vi "Can Edit Cell.vi"(0 "State":T1, 7 "Cell":T6, 11 "NumRows":i32) -> (4 "locked":bool, 8 "can edit?":bool)   [LabVIEW 2020, in "KTable.xctl"]
uses:
  KTable.xctl
  <vilib>/Utility/miscctls.llb/LVRowAndColumnTypeDef.ctl
  State.ctl
  ColumnSpec.ctl
  ColumnType.ctl
  Table Properties.ctl
  Events.ctl
  Event Data.ctl
  Event Type.ctl
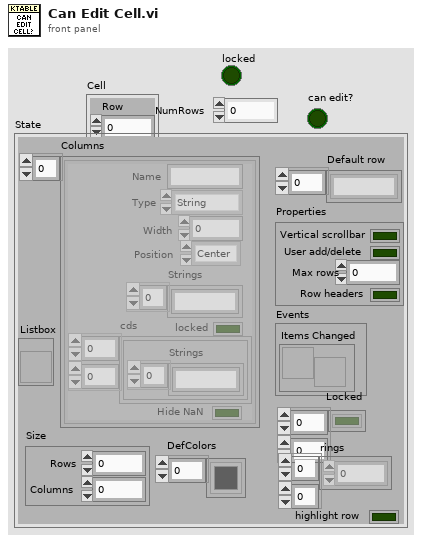
[diagram p1: front panel]
types:
  T1 = typedef "KTable.xctl/State.ctl" = cluster{"Columns":T2[], "Listbox":refnum<vi>, "Default row":string[], "Properties":T4, "Events":T5, "Locked":bool[][], "Size":cluster{"Rows":i32, "Columns":i32}, "rings":i32[][], "DefColors":u32[], "highlight row":bool}
  T2 = typedef "KTable.xctl/ColumnSpec.ctl" = cluster{"Name":string, "Type":T3, "Width":i32, "Strings":string[], "Position":enum16{"Left", "Center", "Right"}, "locked":bool, "cds":cluster{"Strings":string[]}[][], "Hide NaN":bool}
  T3 = typedef "KTable.xctl/ColumnType.ctl" = enum16{"String", "Enum", "Int", "Double", "Boolean", "Ring", "Formula", "Color"}
  T4 = typedef "KTable.xctl/Table Properties.ctl" = cluster{"Vertical scrollbar":bool, "User add/delete":bool, "Max rows":i32, "Row headers":bool}
  T5 = typedef "KTable.xctl/Events.ctl" = cluster{"Items Changed":refnum<user-event>}
  T6 = typedef "LVRowAndColumnTypeDef.ctl" = cluster{"Row":i32, "Column":i32}
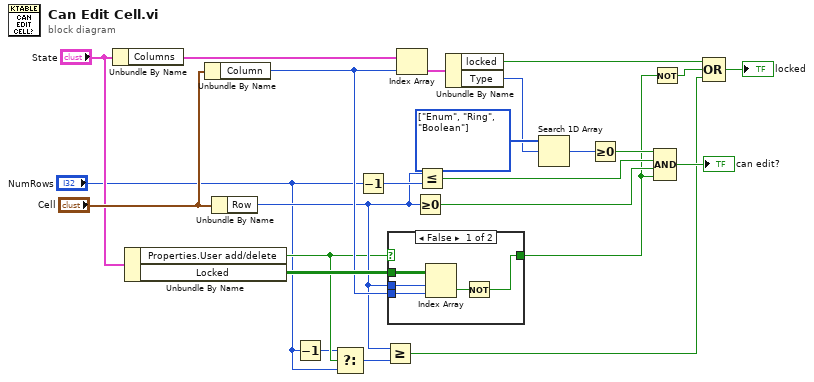
[diagram p0: block diagram]
diagram:
  w23 = T3[] [enum."Enum", enum."Ring", enum."Boolean"] items=["String", "Enum", "Int", "Double", "Boolean", "Ring", "Formula", "Color"] ("y")
  n1 = Unbundle By Name("State") -> ("Columns"=w17:T2[])
  n2 = Unbundle By Name("State") -> ("Properties.User add/delete"=w4:bool, "Locked"=w13:bool[][])
  n3 = Unbundle By Name("Cell") -> ("Column"=w12:i32)
  n4 = Unbundle By Name("Cell") -> ("Row"=w5:i32)
  n5 = Decrement(x="NumRows") -> (x-1=w2:i32)
  n6 = Select(t=w2, s=w4, f="NumRows") -> (s? t:f=w1:i32)
  n7 = Decrement(x="NumRows") -> (x-1=w11:i32)
  n8 = Greater Or Equal?(x=w5, y=w1) -> (x >= y?=w6:bool)
  n9 = case shown="False" w4 {
    selector: w4 -> [_ w30]
    tunnel: [w25 w30] -> w7
    tunnel: w13 -> [w29 _]
    tunnel: w5 -> [w28 _]
    tunnel: w12 -> [w27 _]
    frame False {
      n10 = Index Array(array=w29, index (row)=w28, index (col)=w27) -> (element=w26:bool)
      n11 = Not(x=w26) -> (.not. x?=w25:bool)
    }
    frame True {
    }
  }
  n12 = Index Array(array=w17, index=w12) -> (element=w24:T2)
  n13 = Greater Or Equal To 0?(x=w5) -> (x >= 0?=w20:bool)
  n14 = Less Or Equal?(x=w5, y=w11) -> (x <= y?=w19:bool)
  n15 = Unbundle By Name(w24) -> ("locked"=w10:bool, "Type"=w18:T3)
  n16 = Search 1D Array(1D array=w23, element=w18) -> (index of element=w22:i32)  [unwired: 1 in]
  n17 = Greater Or Equal To 0?(x=w22) -> (x >= 0?=w21:bool)
  n18 = Not(x=w7) -> (.not. x?=w8:bool)
  n19 = Compound Arithmetic op=AND(w21, w19, w20, w7) -> (→"can edit?":bool)
  n20 = Compound Arithmetic op=OR(w10, w8, w6) -> (→"locked":bool)
